vi "PID closed_loop.vi"() -> ()   [LabVIEW 2018]
panel:
  out "magnet_input_pr":dbl
  out "magnet_input_dr":dbl
  in  "desired_relative_y":dbl=754.275
  in  "desired_relative_x":dbl=129.0
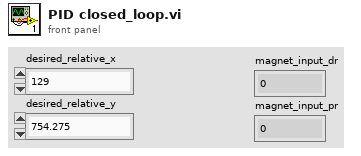
[diagram p1: front panel]
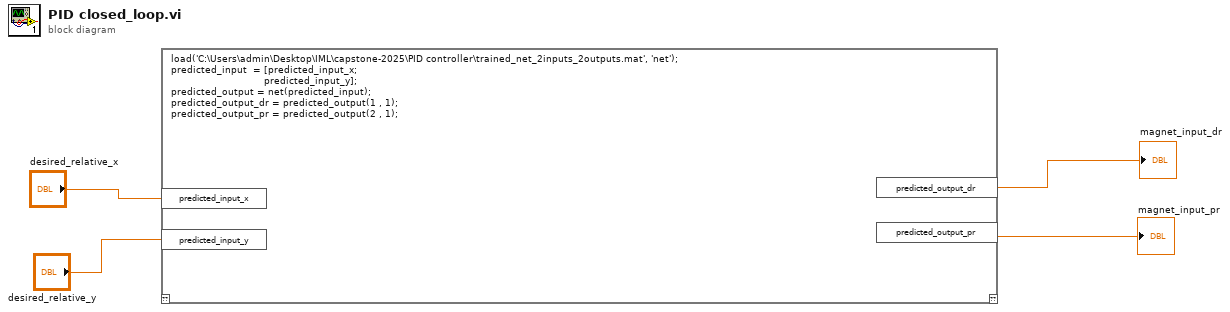
[diagram p0: block diagram]
diagram:
  n1 = script code="load('C:\\Users\\admin\\Desktop\\IML\\capstone-2025\\PID controller\\trained_net_2inputs_2outputs.mat', 'net');\npredicted_input  = [predicted_input_x; \n                               predicted_input_y];\npredicted_output = net(predicted_input);\npredicted_output_dr = predicted_output(1 , 1);\npredicted_output_pr = predicted_output(2 , 1);"("predicted_input_y"="desired_relative_y", "predicted_input_x"="desired_relative_x") -> ("predicted_output_dr"=→"magnet_input_dr":dbl, "predicted_output_pr"=→"magnet_input_pr":dbl)  [unwired: 1 in, 1 out]
